vi "AVS_Init.vi"(9 "a_Port":i32) -> (10 "Output Value":i32)   [LabVIEW 2020]
uses:
  AvaSpecX64-DLL_9.4/avaspecx64.dll
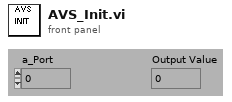
[diagram p1: front panel]
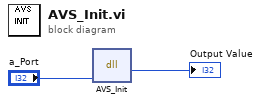
[diagram p0: block diagram]
diagram:
  n1 = dll-call lib="C:/AvaSpecX64-DLL_9.4/avaspecx64.dll" fn="AVS_Init"("a_Port"="a_Port") -> ("return type"=→"Output Value":i32)  [unwired: 4 in, 2 out]
